vi "HandleLowGoal.vi"(7 "InitState":T1, 8 "error in":errorcluster, 11 "Toggle?":bool) -> (0 "error out":errorcluster, 3 "ShootState":T1)   [LabVIEW 2015]
doc: "On First Call:\nIf Toggle then Shoot:\n Else Stop\nAfter First Call:\nIf Toggle then Stop:\n Else Previous Value in Shift Register"
uses:
  LowGoalState.ctl
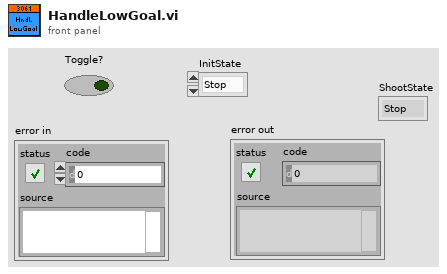
[diagram p1: front panel]
types:
  T1 = typedef "LowGoalState.ctl" = enum16{"Stop", "Shoot"}
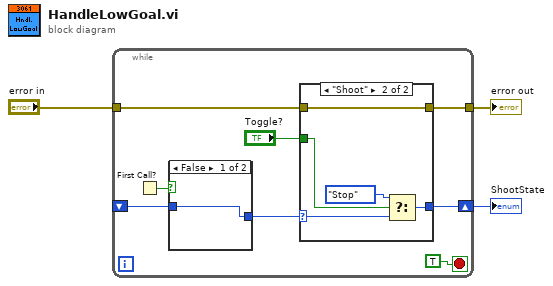
[diagram p0: block diagram]
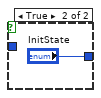
[diagram p2: hidden frame]
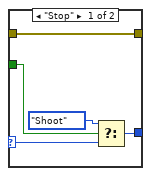
[diagram p3: hidden frame]
diagram:
  n1 = while {
    tunnel: "error in" -> [w9]
    tunnel: [w8] -> w2
    shift-right: [w5] -> w1
    shift-left: _ -> [w4]
    stop <- TRUE stop-if-true
    n2 = First Call?() -> (First Call?: T/F=w10:bool)
    n3 = case shown="False" w10 {
      tunnel: [w12 "InitState"] -> w6
      tunnel: w4 -> [w12 _]
      frame False {
      }
      frame True {
      }
    }
    n4 = case shown="\"Shoot\"" w6 {
      selector: w6 -> [w17 w22]
      tunnel: w9 -> [w18 w19]
      tunnel: [w18 w19] -> w8
      tunnel: [w16 w20] -> w5
      tunnel: "Toggle?" -> [w15 w21]
      frame "Stop" {
        n5 = Select(t=LowGoalState."Shoot" ("InitState 2"), s=w15, f=w17) -> (s? t:f=w16:T1)
      }
      frame "Shoot" {
        n6 = Select(t=LowGoalState."Stop" ("InitState 2"), s=w21, f=w22) -> (s? t:f=w20:T1)
      }
    }
  }
  "error out" <- w2
  "ShootState" <- w1
